vi "Acquisition & Generation test UI.vi"() -> ()   [LabVIEW 2014]
uses:
  <vilib>/FPGAPlugInAG/sbRIO-9636/niLvFpga_Open_sbRIO-9636.vi
  <vilib>/rvi/interface/common/dynamic/niFpgaDynamicAddResources.vi
  <vilib>/rvi/interface/common/niFpgaWaitOnOcc.vi
  <vilib>/Utility/error.llb/Error Cluster From Error Code.vi
  <vilib>/FPGAPlugInAG/Dynamic/niLvFpga_Run_Dynamic.vi
  <vilib>/rvi/errors/niLvFpgaAdjustHostInterfaceError.vi
  <vilib>/FPGAPlugInAG/Dynamic/niLvFpga_Close_Dynamic.vi
  <vilib>/rvi/interface/nirviOpenFPGA/nirviOpenFPGA.xnode
  FPGA Bitfiles/LaserDistanceSen_FPGATarget_Acquisition&Gene_-NqtJmKGZ+s.lvbitx
  FPGA Target/Test VIs/Acquisition & Generation (Init Memory) test.vi
  <vilib>/rvi/interface/nirviMethod/nirviMethod.xnode
  <vilib>/rvi/interface/nirviCloseFPGA/nirviCloseFPGA.xnode
  <vilib>/rvi/errors/niLvFpgaMergeErrorWithErrorCode.vi
  <vilib>/FPGAPlugInAG/Dynamic/niLvFpga_ConfigureFifo_Dynamic.vi
  <vilib>/FPGAPlugInAG/Dynamic/niLvFpga_StartFifo_Dynamic.vi
  <vilib>/FPGAPlugInAG/Dynamic/niLvFpga_ReadFifo_Dynamic.vi
panel:
  out "Waveform Graph":dbl[](graph)
  out "Elements Remaining":u32
  in  "stop":bool
  in  "Number of Elements to read":u32=512
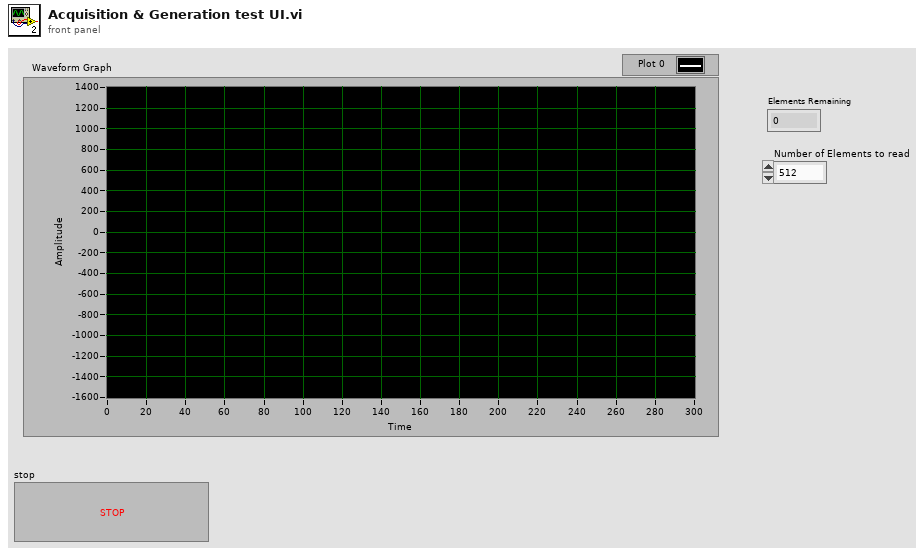
[diagram p1: front panel]
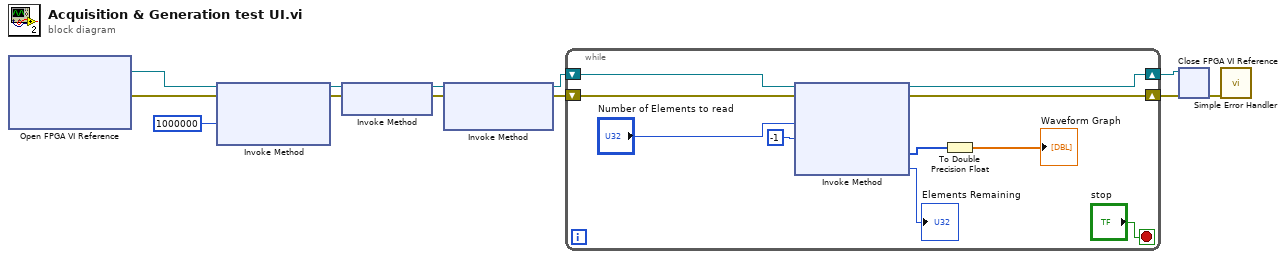
[diagram p0: block diagram]
diagram:
  n1 = xnode "Open FPGA VI Reference"() -> ("FPGA VI Reference Out"=w12:refnum<k20>, "error out"=w11:errorcluster)  [unwired: 2 in]
  n2 = xnode "Invoke Method"("FPGA VI Reference In"=w12, "error in"=w11, "Requested Depth"=u32 1000000) -> ("FPGA VI Reference Out"=w8:refnum<k20>, "error out"=w9:errorcluster)  [unwired: 1 out]
  n3 = xnode "Invoke Method"("FPGA VI Reference In"=w8, "error in"=w9) -> ("FPGA VI Reference Out"=w6:refnum<k20>, "error out"=w7:errorcluster)
  n4 = xnode "Invoke Method"("FPGA VI Reference In"=w6, "error in"=w7) -> ("FPGA VI Reference Out"=w5:refnum<k20>, "error out"=w4:errorcluster)  [unwired: 1 in]
  n5 = while {
    shift-right: [w16] -> w2
    shift-left: w5 -> [w20]
    shift-right: [w15] -> w1
    shift-left: w4 -> [w19]
    stop <- "stop" stop-if-true
    n6 = xnode "Invoke Method"("FPGA VI Reference In"=w20, "error in"=w19, "Number of Elements"="Number of Elements to read", "Timeout (ms)"=-1) -> ("FPGA VI Reference Out"=w16:refnum<k20>, "error out"=w15:errorcluster, "Data"=w14:i16[], "Elements Remaining"=→"Elements Remaining":u32)
    n7 = To Double Precision Float(number=w14) -> (double precision float=→"Waveform Graph":dbl[])
  }
  n8 = xnode "Close FPGA VI Reference"("FPGA VI Reference In"=w2, "error in"=w1) -> ("error out"=w3:errorcluster)
  n9 = call <vilib>:"Simple Error Handler.vi"("error in (no error)"=w3) -> ()  [unwired: 4 in, 5 out]
